vi "ConfigureDlg.vi"(8 "error in (no error)":errorcluster, 11 "StateFunction in":refnum<class "StateFunction.lvclass">) -> (0 "error out":errorcluster, 2 "Changed":bool, 3 "StateFunction out":refnum<class "StateFunction.lvclass">)   [LabVIEW 2014, in "StateFunction.lvclass"]
uses:
  StateFunction.lvclass
  ArbitraryFunction/TypeDefs/Arbitrary.ctl
  ArbitraryFunction/ArbitraryFunction.lvclass
panel:
  in  "Arbs":T1[](array[typedef])
  in  "SampleRate":dbl
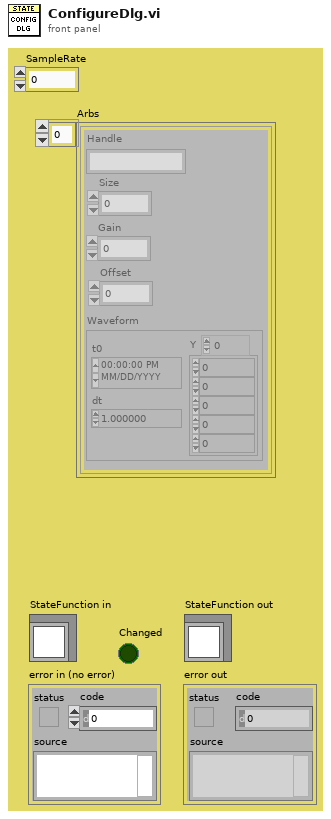
[diagram p1: front panel]
types:
  T1 = typedef "Functions.lvlib/ArbitraryFunction.lvclass/Arbitrary.ctl" = cluster{"Handle":string, "Size":i32, "Gain":dbl, "Offset":dbl, "Waveform":waveform(dbl)}
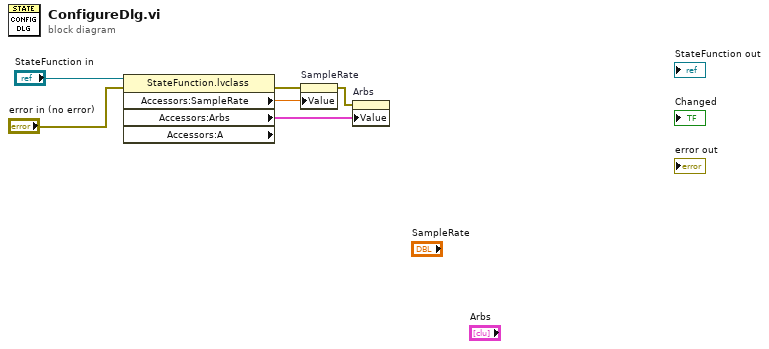
[diagram p0: block diagram]
diagram:
  n1 = property class="StateFunction.lvclass" props=["Accessors:SampleRate", "Accessors:Arbs", "Accessors:A"](reference="StateFunction in", error in="error in (no error)") -> (error out=w4:errorcluster, "Accessors:SampleRate"=w3:dbl, "Accessors:Arbs"=w2:T1[])  [unwired: 2 out]
  n2 = property on="SampleRate" class="DigNum (strict)"(error in=w4, "Value"=w3) -> (error out=w1:errorcluster)  [unwired: 1 in, 1 out]
  n3 = property on="Arbs" class="Arr (strict)"(error in=w1, "Value"=w2) -> ()  [unwired: 1 in, 2 out]
